vi "Enqueue Data To Nodes.vi"(8 "error in":errorcluster, 9 "Input Valid":bool, 10 "Input Data":T1, 11 "Communication FIFOs":T2) -> (0 "error out":errorcluster, 1 "Send Success?":bool, 4 "Ready for Input":bool)   [LabVIEW 2014, in "IO Node Logic Template_SPIBus0.lvlib"]
uses:
  IO Node Logic Template_SPIBus0.lvlib
  Controls/All Nodes Resources.ctl
  Node/Controls/NodeResources FIFOs.ctl
  <vilib>/SPIAPI/Controls/SPI Response Information.ctl
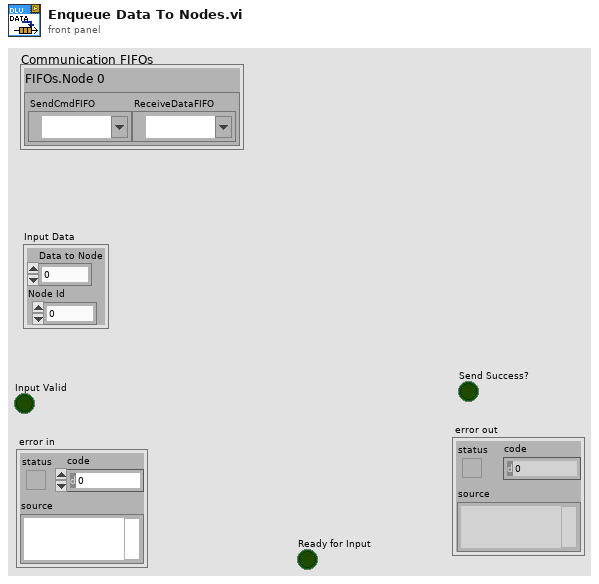
[diagram p1: front panel]
types:
  T1 = typedef "SPI Response Information.ctl" = cluster{"Data to Node":u64, "Node Id":u16}
  T2 = typedef "IO Node Logic Template_SPIBus0.lvlib/All Nodes Resources.ctl" = cluster{"FIFOs.Node 0":T3}
  T3 = typedef "IO Node Logic Template_SPIBus0.lvlib/NodeResources FIFOs.ctl" = cluster{"SendCmdFIFO":refnum<k21>, "ReceiveDataFIFO":refnum<k21>}
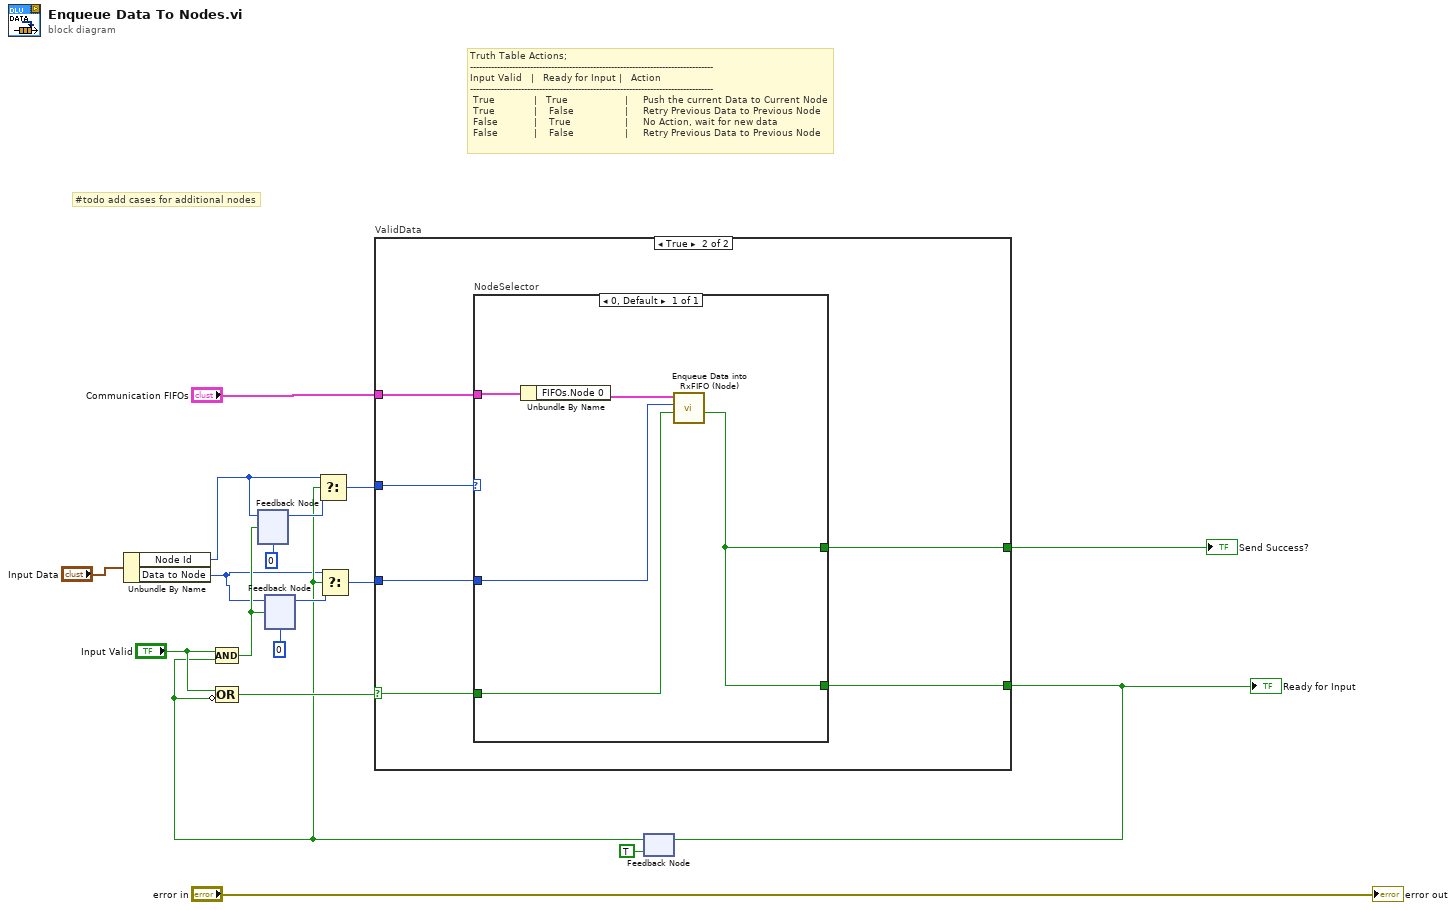
[diagram p0: block diagram]
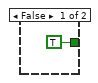
[diagram p2: hidden frame]
diagram:
  # "#todo add cases for additional nodes"
  # "Truth Table Actions;\n---------------------------------------------------------------------------------\nInput Valid   |   Ready for Input |   Action\n---------------------------------------------------------------------------------\n True             |   True                   |     Push the current Data to Current Node\n True             |    False                 |     Retry Previous Data to Previous Node\n False            |    True                  |     No Action, wait for new data\n False            |    False                 |     Retry Previous Data to Previous Node"
  n1 = Unbundle By Name("Input Data") -> ("Node Id"=w1:u16, "Data to Node"=w2:u64)
  n2 = feedback #1(u8 0 ("Current Node")) -> (w11:u16)
  n3 = feedback #2(u64 0 ("Input Data")) -> (w9:u64)
  n4 = feedback #3(TRUE ("Send Success?")) -> (w7:bool)
  n5 = Compound Arithmetic op=AND("Input Valid", w7) -> (w15:bool)
  n6 = Compound Arithmetic op=OR("Input Valid", invert w7) -> (w13:bool)
  n7 = feedback-in #1(w1, w15) -> ()
  n8 = feedback-in #2(w2, w15) -> ()
  n9 = Select(t=w1, s=w7, f=w11) -> (s? t:f=w12:u16)
  n10 = Select(t=w2, s=w7, f=w9) -> (s? t:f=w10:u64)
  n11 = case "ValidData" shown="True" w13 {
    selector: w13 -> [_ w22]
    tunnel: "Communication FIFOs" -> [_ w25]
    tunnel: w12 -> [_ w24]
    tunnel: w10 -> [_ w23]
    tunnel: [TRUE ("Send Success?") w21] -> w16
    tunnel: [_ w20] -> w3
    frame False {
    }
    frame True {
      n12 = case "NodeSelector" shown="0, Default" w24 {
        tunnel: w25 -> [w30]
        tunnel: w23 -> [w28]
        tunnel: w22 -> [w27]
        tunnel: [w26] -> w21
        tunnel: [w26] -> w20
        frame 0, Default {
          n13 = Unbundle By Name(w30) -> ("FIFOs.Node 0"=w29:T3)
          n14 = call "Enqueue Data into RxFIFO (Node).vi"("Input Valid"=w27, "Input Data"=w28, "FIFOs: I/O Node"=w29) -> ("Send Success?"=w26:bool)  [unwired: 6 in, 2 out]
        }
      }
    }
  }
  "Ready for Input" <- w16
  "Send Success?" <- w3
  n15 = feedback-in #3(w16) -> ()
  "error out" <- "error in"
